vi "biquad_fxp.vi"(7 "reset":bool=TRUE, 8 "input valid":bool=TRUE, 11 "x":fxp<+/-,32,14>) -> (0 "output valid":bool, 3 "y":fxp<+/-,32,14>)   [LabVIEW 2018]
doc: "One second order section, Direct form 1\nRequires 10 cycles per actual sample"
uses:
  <vilib>/rvi/Emulation/niFpgaEmulationIsFPGAContextNoSignature.vi
  <vilib>/rvi/DataTransferAndStorage/Container/Common/niFpgaContainerGetUniqueNameForEmu.vi
  <vilib>/rvi/Memory/Memory_Emulation/niFpgaMemoryEmulationCacheClearOnFirstRun.vi
  <vilib>/rvi/Memory/Memory_Emulation/nirvimemoryEmulationManagerCache_MakeExclusive.vi
  <vilib>/rvi/Memory/Memory_Emulation/niFpgaMemoryEmulationValidateCache.vi
  <vilib>/rvi/Memory/Memory_Emulation/nirvimemoryEmulationManagerCache_InsertValue.vi
  <vilib>/Utility/error.llb/Clear Errors.vi
  <vilib>/rvi/Memory/Memory_Emulation/nirvimemoryEmulationManagerCache_ReleaseExclusive.vi
  <vilib>/rvi/Memory/Memory_Emulation/nirvimemoryEmulationManagerCache_GetValue.vi
  <vilib>/rvi/Memory/Memory_Emulation/nirvimemoryEmulationManagerCache_SetValue.vi
  <vilib>/rvi/Emulation/niFpgaProcessEmulError.vi
  <vilib>/rvi/Emulation/niFpgaSctlEmulationGetInTimedLoop.vi
  <vilib>/rvi/DataTransferAndStorage/Container/XNode/niFpgaContainer.xnode
  <vilib>/rvi/DataTransferAndStorage/Register/Emulation/niFpgaRegisterEmulation.vi
  <vilib>/rvi/FXPMathLib/FxpMul/XNode/nifxpmath_Multiplier.xnode
  <vilib>/rvi/FXPMathLib/FxpAdd/XNode/nifxpmath_Add.xnode
  <vilib>/rvi/FXPMathLib/sim/FxpSim.dll
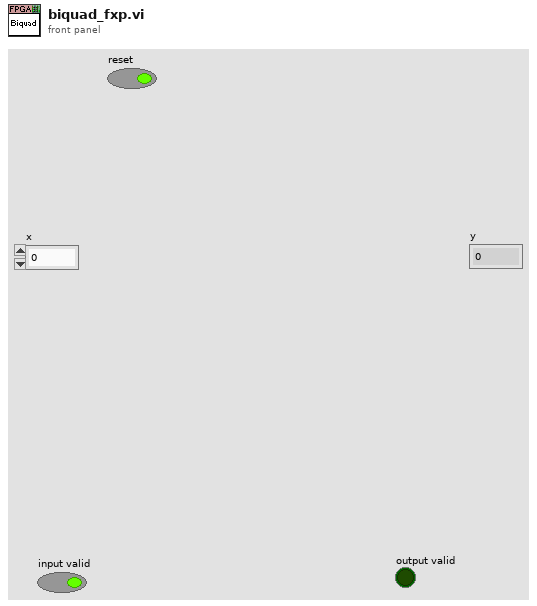
[diagram p1: front panel]
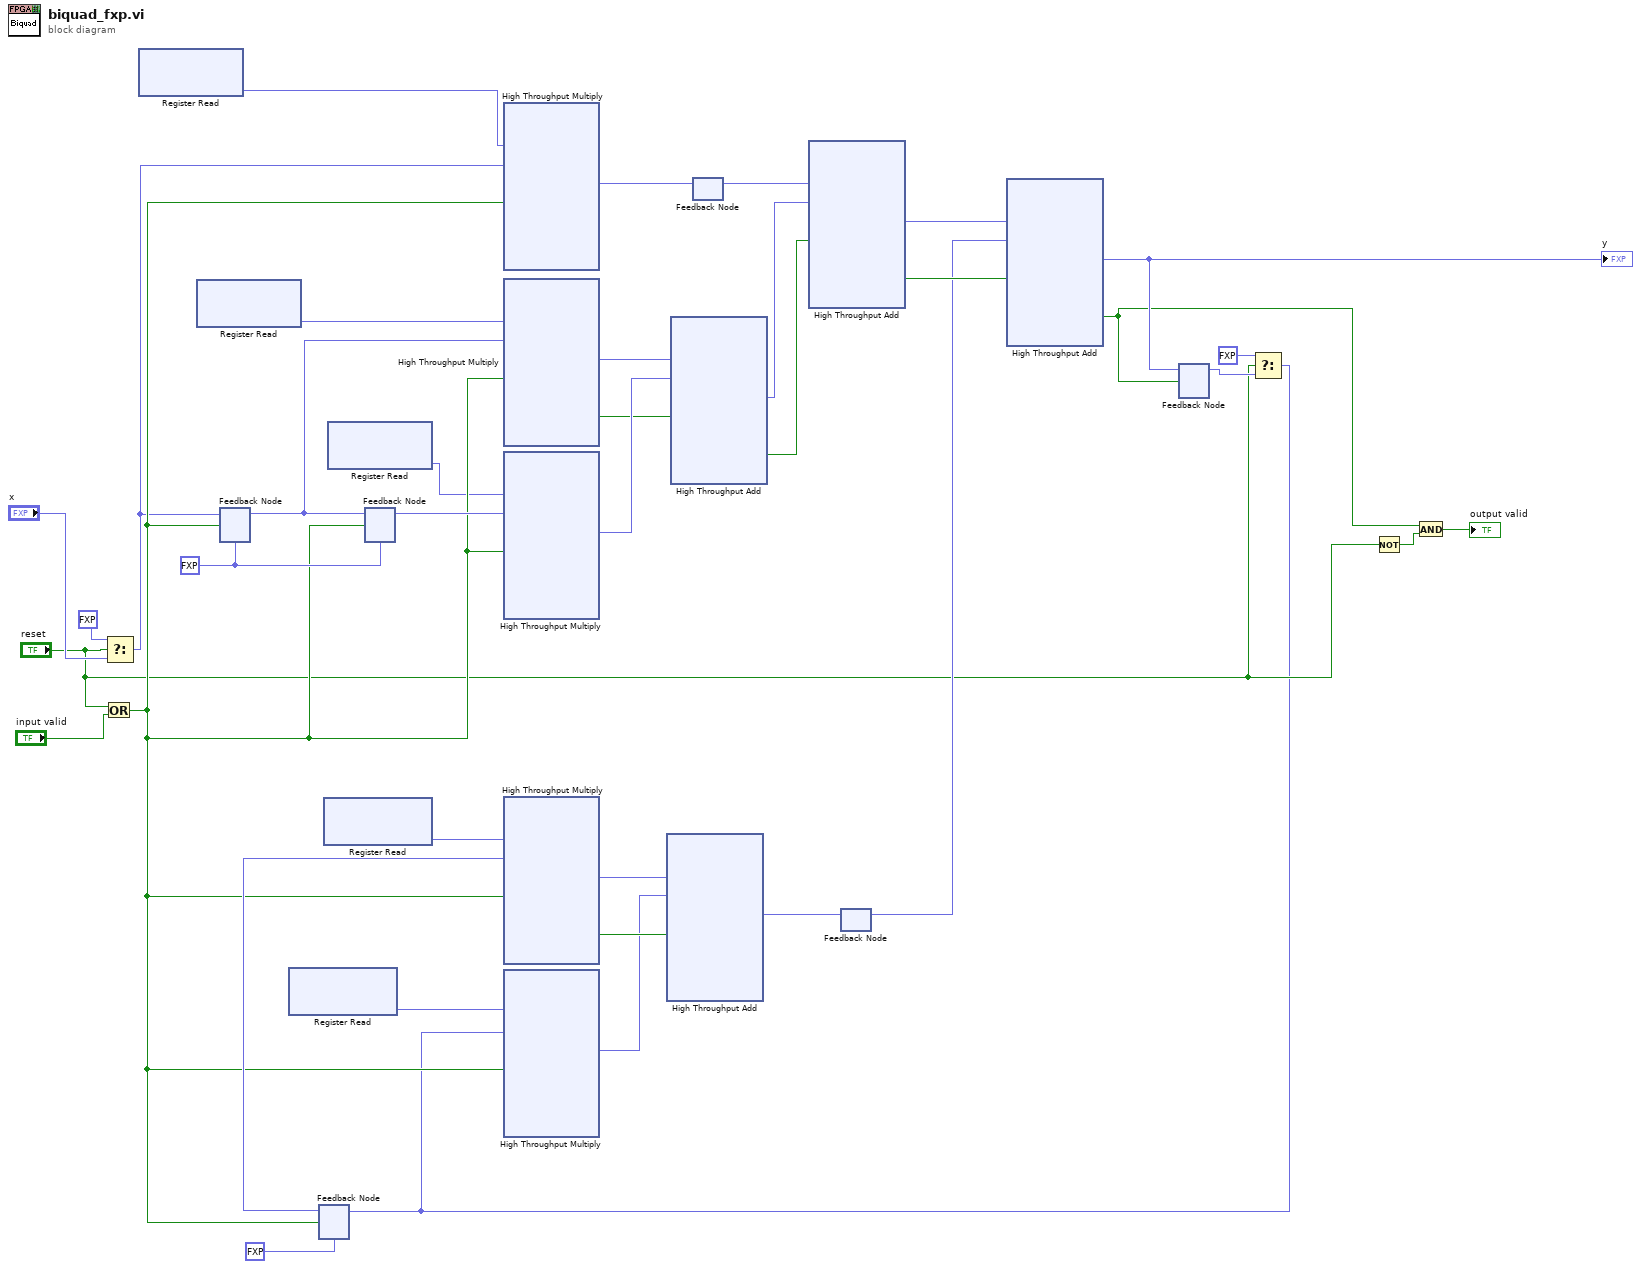
[diagram p0: block diagram]
diagram:
  w21 = fxp<+/-,32,14> 0.0 ("x")
  n1 = Or(x="reset", y="input valid") -> (x .or. y?=w14:bool)
  n2 = Select(t=fxp<+/-,32,14> 0.0 ("x"), s="reset", f="x") -> (s? t:f=w10:fxp<+/-,32,14>)
  n3 = xnode "Register Read"() -> ("Data"=w5:fxp<+/-,32,2>)  [unwired: 1 in, 1 out]
  n4 = xnode "Register Read"() -> ("Data"=w4:fxp<+/-,32,2>)  [unwired: 1 in, 1 out]
  n5 = feedback #1(w21) -> (w37:fxp<+/-,32,14>)
  n6 = feedback-in #1(w10, w14) -> ()
  n7 = xnode "Register Read"() -> ("Data"=w1:fxp<+/-,32,2>)  [unwired: 1 in, 1 out]
  n8 = feedback #2(fxp<+/-,32,14> 0.0 ("x")) -> (w30:fxp<+/-,32,14>)
  n9 = xnode "Register Read"() -> ("Data"=w2:fxp<+/-,32,2>)  [unwired: 1 in, 1 out]
  n10 = xnode "Register Read"() -> ("Data"=w3:fxp<+/-,32,2>)  [unwired: 1 in, 1 out]
  n11 = feedback #3(w21) -> (w36:fxp<+/-,32,14>)
  n12 = feedback-in #3(w37, w14) -> ()
  n13 = xnode ("High Throughput Multiply")("x"=w5, "y"=w10, "input valid"=w14) -> ("x*y"=w24:fxp<+/-,32,14>)  [unwired: 1 in, 2 out]
  n14 = xnode ("High Throughput Multiply")("x"=w4, "y"=w37, "input valid"=w14) -> ("x*y"=w35:fxp<+/-,32,14>, "output valid"=w33:bool)  [unwired: 1 in, 1 out]
  n15 = xnode ("High Throughput Multiply")("x"=w3, "y"=w36, "input valid"=w14) -> ("x*y"=w34:fxp<+/-,32,14>)  [unwired: 1 in, 2 out]
  n16 = xnode ("High Throughput Multiply")("x"=w2, "y"=w30, "input valid"=w14) -> ("x*y"=w29:fxp<+/-,32,14>, "output valid"=w28:bool)  [unwired: 1 in, 1 out]
  n17 = xnode "High Throughput Add"("x"=w35, "y"=w34, "input valid"=w33) -> ("x+y"=w32:fxp<+/-,32,14>, "output valid"=w31:bool)  [unwired: 1 in, 1 out]
  n18 = feedback-in #4(w24) -> ()
  n19 = feedback #4() -> (w23:fxp<+/-,32,14>)  [unwired: 1 in]
  n20 = xnode "High Throughput Add"("x"=w23, "y"=w32, "input valid"=w31) -> ("x+y"=w26:fxp<+/-,32,14>, "output valid"=w25:bool)  [unwired: 1 in, 1 out]
  n21 = feedback #5() -> (w18:fxp<+/-,32,14>)  [unwired: 1 in]
  n22 = xnode "High Throughput Add"("x"=w26, "y"=w18, "input valid"=w25) -> ("x+y"=w19:fxp<+/-,32,14>, "output valid"=w13:bool)  [unwired: 1 in, 1 out]
  "y" <- w19
  n23 = feedback #6() -> (w9:fxp<+/-,32,14>)  [unwired: 1 in]
  n24 = feedback-in #6(w19, w13) -> ()
  n25 = Select(t=fxp<+/-,32,14> 0.0, s="reset", f=w9) -> (s? t:f=w6:fxp<+/-,32,14>)
  n26 = feedback-in #2(w6, w14) -> ()
  n27 = xnode ("High Throughput Multiply")("x"=w1, "y"=w6, "input valid"=w14) -> ("x*y"=w27:fxp<+/-,32,14>)  [unwired: 1 in, 2 out]
  n28 = xnode "High Throughput Add"("x"=w29, "y"=w27, "input valid"=w28) -> ("x+y"=w22:fxp<+/-,32,14>)  [unwired: 1 in, 2 out]
  n29 = feedback-in #5(w22) -> ()
  n30 = Not(x="reset") -> (.not. x?=w12:bool)
  n31 = And(x=w13, y=w12) -> (x .and. y?=→"output valid":bool)
